vi "DeQueue.vi"(7 "QueName":string="BaseVisQue", 8 "Error":errorcluster[](array[cluster])) -> (0 "Error":errorcluster[](array[cluster]), 1 "Data":variant, 2 "Message":string)   [LabVIEW 2014, in "Visualization.lvlib" / "VisualizeBase.lvclass"]
uses:
  VisualizeBase/VisualizeBase_class/VisualizeBase.lvclass
  Typedefs/MsgType.ctl
  <userlib>/NIST/NISTErrorLib/NISTErrorLib.lvlib
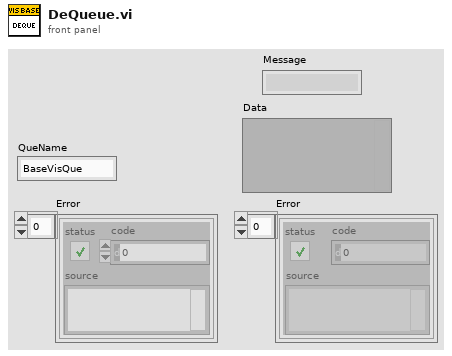
[diagram p1: front panel]
types:
  T1 = typedef "Visualization.lvlib/VisualizeBase.lvclass/MsgType.ctl" = cluster{"Message":string, "Data":variant}
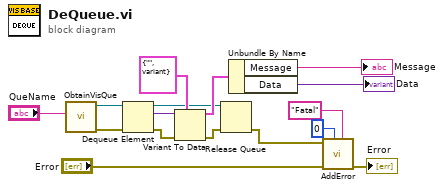
[diagram p0: block diagram]
diagram:
  n1 = call "ObtainVisQue.vi"("QueName"="QueName") -> ("error out"=w15:errorcluster, "queue out"=w16:refnum<queue>)  [unwired: 9 in]
  n2 = Dequeue Element(queue=w16, error in (no error)=w15) -> (queue out=w3:refnum<queue>, element=w14:variant, error out=w13:errorcluster)  [unwired: 1 in, 1 out]
  n3 = Variant To Data(error in=w13, type=T1 {"Message"="", "Data"=variant} ("clMsgType"), Variant=w14) -> (data=w11:T1, error out=w2:errorcluster)
  n4 = Release Queue(queue=w3, error in (no error)=w2) -> (error out=w1:errorcluster)  [unwired: 1 in, 2 out]
  n5 = Unbundle By Name(w11) -> ("Message"=→"Message":string, "Data"=→"Data":variant)
  n6 = call <userlib>:"AddError.vi"("Severity"="Fatal" ("String"), "Priority"=u8 0, "ErrorArray"="Error", "error in (no error)"=w1) -> ("ErrorArray"=→"Error":errorcluster[])  [unwired: 6 in, 1 out]
